vi "Presynthesize.vi"(0 "FM Sweep in":refnum<class "FM Sweep.lvclass">, 5 "Channel in":refnum<class "Channel.lvclass">, 11 "error in (no error)":errorcluster) -> (4 "FM Sweep out":refnum<class "FM Sweep.lvclass">, 6 "Channel out":refnum<class "Channel.lvclass">, 15 "error out":errorcluster)   [LabVIEW 2020, in "FM Sweep.lvclass"]
uses:
  FM Sweep.lvclass
  Channel/Channel.lvclass
  FM Sweep.lvclass/FM Sweep.ctl
  Channel/Channel.lvclass/Channel.ctl
  Gate/Gate.lvclass/Gate.ctl
  Channel/Read Gate.vi
  Gate/Read Ramp (ms).vi
  Gate/Write Duration (ms).vi
  Channel/Write Gate.vi
  Gate/Gate.lvclass
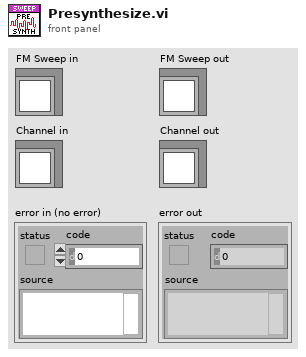
[diagram p1: front panel]
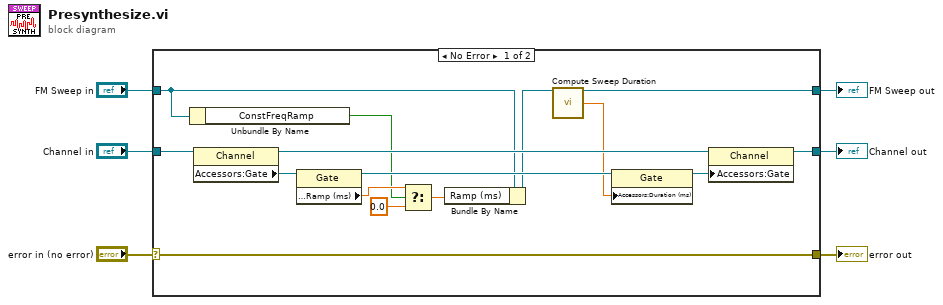
[diagram p0: block diagram]
diagram:
  n1 = case shown="No Error" "error in (no error)" {
    selector: "error in (no error)" -> [w21 w22]
    tunnel: "FM Sweep in" -> [w11 w24]
    tunnel: [w13 w24] -> w4
    tunnel: [w15 w23] -> w3
    tunnel: "Channel in" -> [w20 w23]
    tunnel: [w21 w22] -> w1
    frame No Error {
      n2 = Unbundle By Name(w11) -> ("ConstFreqRamp"=w9:bool)
      n3 = property class="Channel"(reference=w20) -> (reference out=w17:refnum<class "Channel.lvclass">, "Accessors:Gate"=w19:refnum<class "Gate.lvclass">)  [unwired: 1 in, 1 out]
      n4 = property class="Gate"(reference=w19) -> (reference out=w18:refnum<class "Gate.lvclass">, "Accessors:Ramp (ms)"=w10:dbl)  [unwired: 1 in, 1 out]
      n5 = Select(t=w10, s=w9, f=0.0) -> (s? t:f=w8:dbl)
      n6 = Bundle By Name(cluster=w11, "Ramp (ms)"=w8) -> (w14:refnum<class "FM Sweep.lvclass">)
      n7 = call "Compute Sweep Duration.vi"("FM Sweep in"=w14) -> ("FM Sweep out"=w13:refnum<class "FM Sweep.lvclass">, "Duration (ms)"=w12:dbl)  [unwired: 12 in, 1 out]
      n8 = property class="Gate"(reference=w18, "Accessors:Duration (ms)"=w12) -> (reference out=w16:refnum<class "Gate.lvclass">)  [unwired: 1 in, 1 out]
      n9 = property class="Channel"(reference=w17, "Accessors:Gate"=w16) -> (reference out=w15:refnum<class "Channel.lvclass">)  [unwired: 1 in, 1 out]
    }
    frame Error {
    }
  }
  "error out" <- w1
  "FM Sweep out" <- w4
  "Channel out" <- w3
